vi "set_readiness.vi"(8 "error in (no error)":errorcluster, 10 "ready?":bool, 11 "DAQ_DL090211Scaffold in":refnum<class "DAQ_DL090211Scaffold.lvclass">) -> (0 "error out":errorcluster, 3 "DAQ_DL090211Scaffold out":refnum<class "DAQ_DL090211Scaffold.lvclass">)   [LabVIEW 2010, in "DAQ_DL090211Scaffold.lvclass"]
uses:
  DAQ_DL090211Scaffold.lvclass
  DAQ_DL090211Scaffold.lvclass/DAQ_DL090211Scaffold.ctl
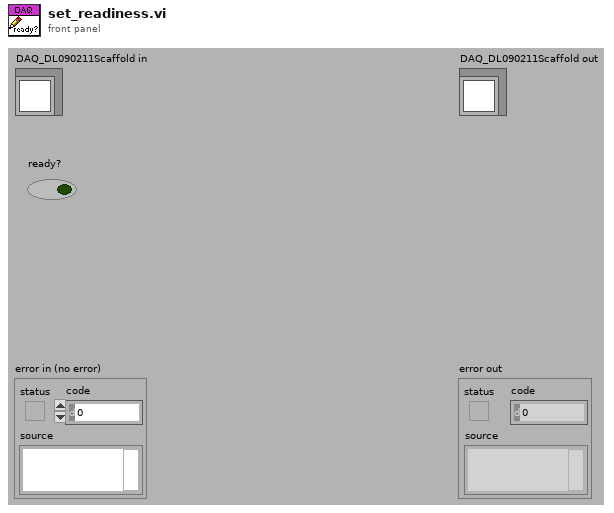
[diagram p1: front panel]
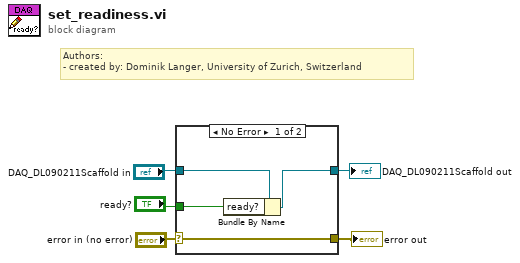
[diagram p0: block diagram]
diagram:
  # "Authors: \n- created by: Dominik Langer, University of Zurich, Switzerland"
  n1 = case shown="No Error" "error in (no error)" {
    selector: "error in (no error)" -> [w9 w11]
    tunnel: [w9 w11] -> w4
    tunnel: [w6 w10] -> w2
    tunnel: "DAQ_DL090211Scaffold in" -> [w7 w10]
    tunnel: "ready?" -> [w8 _]
    frame No Error {
      n2 = Bundle By Name(cluster=w7, "ready?"=w8) -> (w6:refnum<class "DAQ_DL090211Scaffold.lvclass">)
    }
    frame Error {
    }
  }
  "error out" <- w4
  "DAQ_DL090211Scaffold out" <- w2
